vi "ILABs_IsLoaded.vi"(2 "error in (no error)":errorcluster, 3 "appRef":refnum<vi>, 4 "name":string) -> (0 "error out":errorcluster, 1 "status":bool)   [LabVIEW 2009]
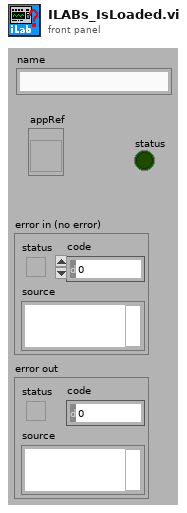
[diagram p1: front panel]
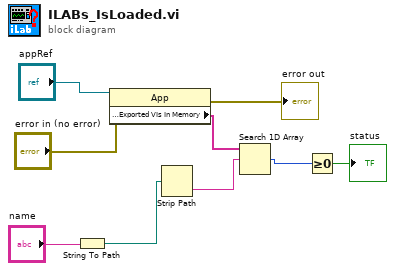
[diagram p0: block diagram]
diagram:
  n1 = String To Path(string="name") -> (path=w2:path)
  n2 = property class="App"(reference="appRef", error in="error in (no error)") -> (error out=→"error out":errorcluster, "Application:Exported VIs In Memory"=w9:string[])  [unwired: 1 out]
  n3 = Strip Path(path=w2) -> (name=w1:string)  [unwired: 1 out]
  n4 = Search 1D Array(1D array=w9, element=w1) -> (index of element=w8:i32)  [unwired: 1 out]
  n5 = Greater Or Equal To 0?(x=w8) -> (x >= 0?=→"status":bool)
